vi "Error Core.vi"(8 "error in (no error)":errorcluster, 10 "String to Append":string, 11 "Error":T1) -> (0 "error out":errorcluster)   [LabVIEW 2021, in "Time_CIF_U.lvlib"]
uses:
  Time_CIF_U.lvlib
  Errors/Errors_CIF_U.lvlib
  Typedef/Errors.ctl
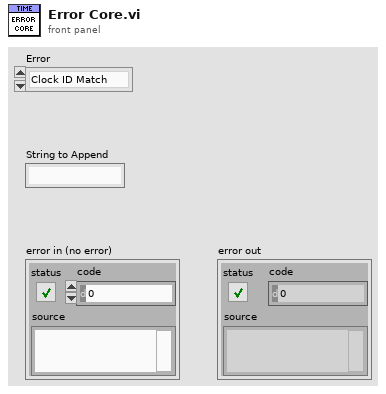
[diagram p1: front panel]
types:
  T1 = typedef "Time_CIF_U.lvlib/Errors.ctl" = enum16{"Clock ID Match", "Invalid Clock ID", "Long Sleep", "Linux Sleep"}
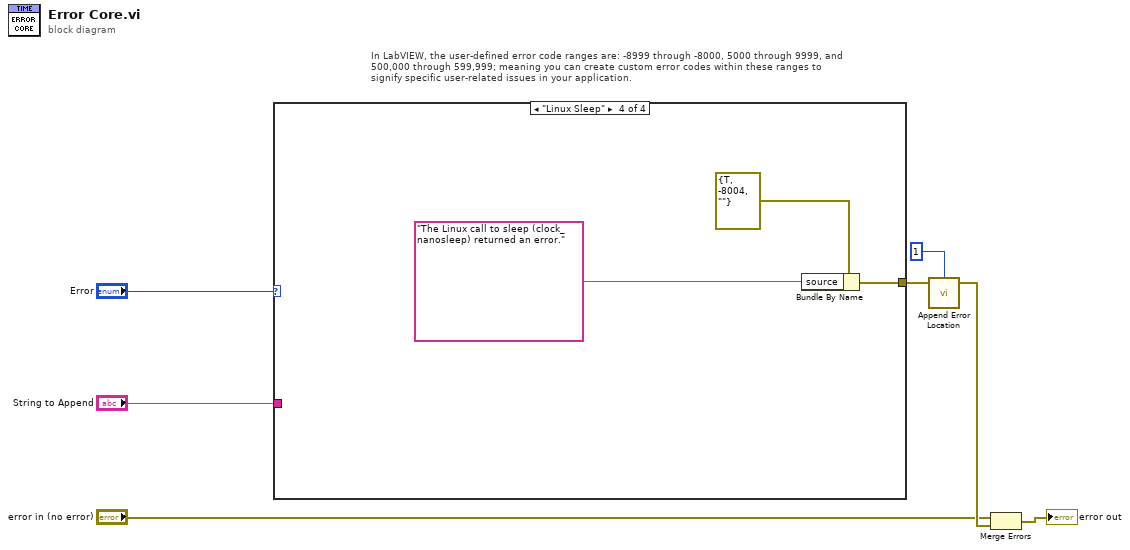
[diagram p0: block diagram]
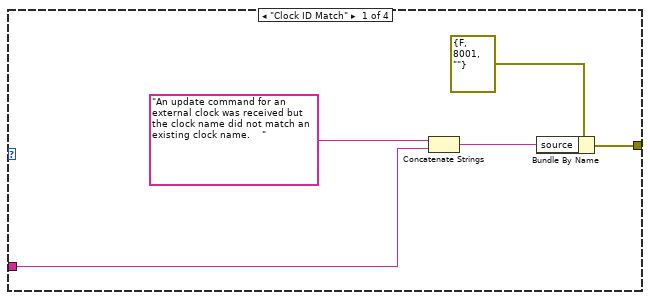
[diagram p2: hidden frame]
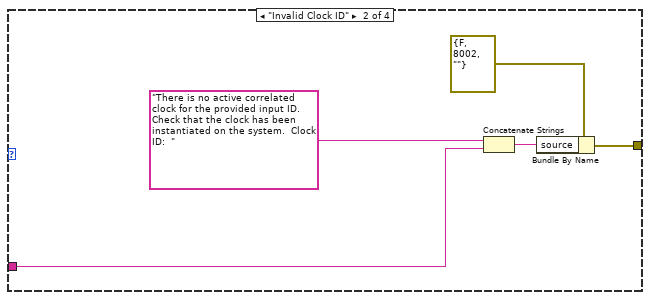
[diagram p3: hidden frame]
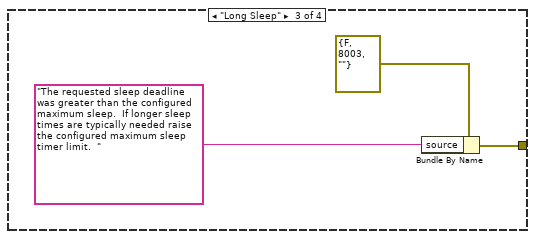
[diagram p4: hidden frame]
diagram:
  # "In LabVIEW, the user-defined error code ranges are: -8999 through -8000, 5000 through 9999, and 500,000 through 599,999; meaning you can create custom error codes within these ranges to signify specific user-related issues in your application."
  n1 = case shown="\"Linux Sleep\"" "Error" {
    tunnel: "String to Append" -> [w8 w14 _ _]
    tunnel: [w11 w16 w19 w22] -> w6
    frame "Clock ID Match" {
      n2 = Concatenate Strings("An update command for an external clock was received but the clock name did not match an existing clock name.    " ("source"), w8) -> (w9:string)
      n3 = Bundle By Name(cluster=errorcluster {"status"=FALSE, "code"=8001, "source"=""} ("Invalid ID"), "source"=w9) -> (w11:errorcluster)
    }
    frame "Invalid Clock ID" {
      n4 = Concatenate Strings("There is no active correlated clock for the provided input ID.  Check that the clock has been instantiated on the system.  Clock ID:  " ("source"), w14) -> (w13:string)
      n5 = Bundle By Name(cluster=errorcluster {"status"=FALSE, "code"=8002, "source"=""} ("Invalid ID"), "source"=w13) -> (w16:errorcluster)
    }
    frame "Long Sleep" {
      n6 = Bundle By Name(cluster=errorcluster {"status"=FALSE, "code"=8003, "source"=""} ("Invalid ID"), "source"="The requested sleep deadline was greater than the configured maximum sleep.  If longer sleep times are typically needed raise the configured maximum sleep timer limit.  ") -> (w19:errorcluster)
    }
    frame "Linux Sleep" {
      n7 = Bundle By Name(cluster=errorcluster {"status"=TRUE, "code"=-8004, "source"=""} ("Invalid ID"), "source"="The Linux call to sleep (clock_nanosleep) returned an error.") -> (w22:errorcluster)
    }
  }
  n8 = call "Append Error Location.vi"("error in (no error)"=w6, "Chain Depth"=1) -> ("error out"=w7:errorcluster)  [unwired: 3 in]
  n9 = Merge Errors("error in (no error)", w7) -> (→"error out":errorcluster)
